vi "Read Stop on Fail_.vi"(8 "error in (no error)":errorcluster, 11 "Assertion Step in":refnum<class "Assertion Step.lvclass">) -> (0 "error out":errorcluster, 2 "Stop on Fail?":bool, 3 "Assertion Step out":refnum<class "Assertion Step.lvclass">)   [LabVIEW 2020, in "MacroAssert.lvlib" / "Assertion Step.lvclass"]
uses:
  Assertion Step.lvclass
  Assertion Step.lvclass/Assertion Step.ctl
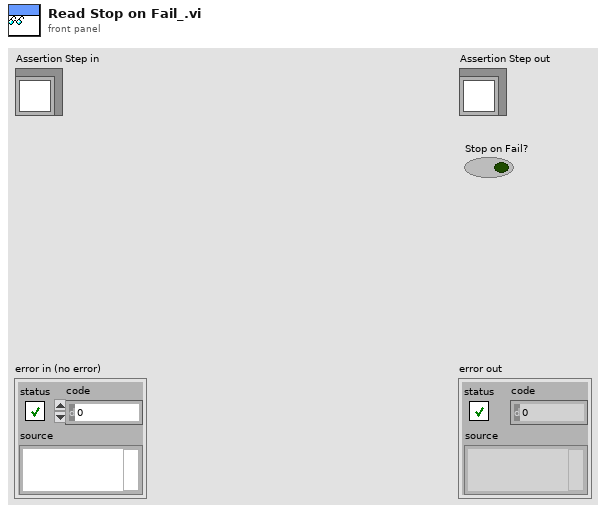
[diagram p1: front panel]
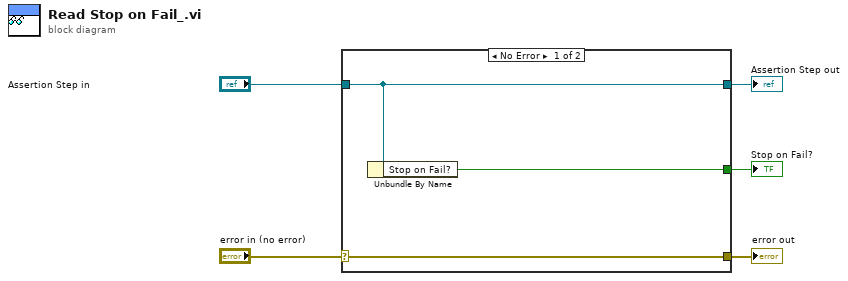
[diagram p0: block diagram]
diagram:
  n1 = case shown="No Error" "error in (no error)" {
    selector: "error in (no error)" -> [w8 w9]
    tunnel: [w8 w9] -> w4
    tunnel: [w7 w10] -> w2
    tunnel: "Assertion Step in" -> [w7 w10]
    tunnel: [w6 _] -> w1
    frame No Error {
      n2 = Unbundle By Name(w7) -> ("Stop on Fail?"=w6:bool)
    }
    frame Error {
    }
  }
  "error out" <- w4
  "Assertion Step out" <- w2
  "Stop on Fail?" <- w1
